vi "HandleTrigger.vi"(8 "error in (no error)":errorcluster, 9 "Current Trigger Value":dbl, 10 "Previous Trigger Value":dbl, 11 "Channel Manager in":refnum<class "Channel Manager.lvclass">) -> (0 "error out":errorcluster, 3 "Channel Manager out":refnum<class "Channel Manager.lvclass">)   [LabVIEW 2024, in "Embedded TDMS Logger Engine.lvlib" / "Channel Manager.lvclass"]
doc: "Overall handler of the trigger, calculates the logic of the trigger state and then if just triggered - opens a new file, if just \"untriggered\", close the file. Log the trigger state and last value for the next stage and iteration.s"
uses:
  Channel Manager.lvclass
  Channel Manager.lvclass/Channel Manager.ctl
  Shared/File Classes/File/File.lvclass
panel:
  out "Just Triggered/Setup?":bool
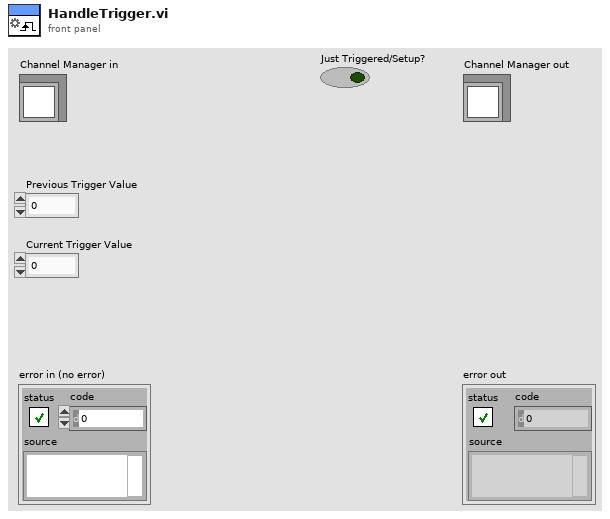
[diagram p1: front panel]
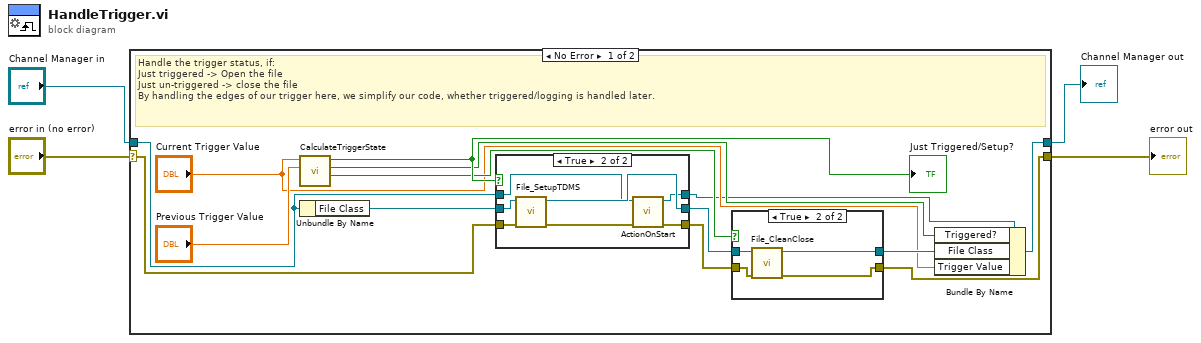
[diagram p0: block diagram]
diagram:
  n1 = case shown="No Error" "error in (no error)" {
    selector: "error in (no error)" -> [w15 w36]
    tunnel: [w9 w36] -> w3
    tunnel: [w13 w35] -> w1
    tunnel: "Channel Manager in" -> [w6 w35]
    frame No Error {
      # "Handle the trigger status, if:\nJust triggered -> Open the file\nJust un-triggered -> close the file\nBy handling the edges of our trigger here, we simplify our code, whether triggered/logging is handled later."
      n2 = call "CalculateTriggerState.vi"("Previous Trigger Value"="Previous Trigger Value", "Current Trigger Value"="Current Trigger Value") -> ("End Triggered/Close?"=w14:bool, "Triggered/Logging?"=w12:bool, "Just Triggered/Setup?"=w17:bool)  [unwired: 7 in]
      "Just Triggered/Setup?" <- w17
      n3 = Unbundle By Name(w6) -> ("File Class"=w16:refnum<class "File.lvclass">)
      n4 = case shown="True" w17 {
        tunnel: w16 -> [w27 w34]
        tunnel: w15 -> [w26 w32]
        tunnel: [w26 w28] -> w11
        tunnel: [w27 w33] -> w10
        tunnel: w6 -> [w25 w31]
        tunnel: [w25 w30] -> w5
        frame False {
        }
        frame True {
          n5 = call-dynamic "File_SetupTDMS.vi"("error in (no error)"=w32, "File in"=w34) -> ("error out"=w29:errorcluster, "File out"=w33:refnum<class "File.lvclass">)  [unwired: 8 in]
          n6 = call-dynamic "ActionOnStart.vi"("error in (no error)"=w29, "Channel Manager in"=w31) -> ("error out"=w28:errorcluster, "Channel Manager out"=w30:refnum<class "Channel Manager.lvclass">)  [unwired: 8 in]
        }
      }
      n7 = case shown="True" w14 {
        tunnel: w11 -> [w20 w23]
        tunnel: w10 -> [w19 w24]
        tunnel: [w20 w22] -> w9
        tunnel: [w19 w21] -> w8
        frame False {
        }
        frame True {
          n8 = call-dynamic "File_CleanClose.vi"("error in (no error)"=w23, "File in"=w24) -> ("error out"=w22:errorcluster, "File out"=w21:refnum<class "File.lvclass">)  [unwired: 8 in]
        }
      }
      n9 = Bundle By Name(cluster=w5, "Triggered?"=w12, "File Class"=w8, "Trigger Value"="Current Trigger Value") -> (w13:refnum<class "Channel Manager.lvclass">)
    }
    frame Error {
    }
  }
  "error out" <- w3
  "Channel Manager out" <- w1
